vi "Actor Core.vi"(8 "error in":errorcluster, 11 "XY WFRM Plot in":refnum<class "XY WFRM Plot.lvclass">) -> (0 "error out":errorcluster, 3 "Actor out":refnum<class "Actor.lvclass">)   [LabVIEW 2020, in "XY WFRM Plot.lvclass"]
doc: "Plots listed TDMS data files"
uses:
  XY WFRM Plot.lvclass
  opt/github/LabActor/Template Module/Template Module.lvclass
  opt/github/LabActor/Plots/Plot/Plot.lvclass
  Applications/National Instruments/LabVIEW 2020 64-bit/vi.lib/ActorFramework/Actor/Actor.lvclass
  <vilib>/ActorFramework/Actor/Actor.lvclass
  Plot types.ctl
  XY WFRM Plot.lvclass/XY WFRM Plot.ctl
  Template Module/Template Module.lvclass/Template Module.ctl
  Plot/Plot.lvclass/Plot.ctl
  <vilib>/ActorFramework/Actor/Actor.lvclass/Actor.ctl
  <vilib>/ActorFramework/Message Enqueuer/Message Enqueuer.lvclass/Message Enqueuer.ctl
  XY WFRM Plot Messages/Set Plot Type Msg/Set Plot Type Msg.lvclass/Set Plot Type Msg.ctl
  Plot Messages/Write Files Msg/Write Files Msg.lvclass/Write Files Msg.ctl
  Plot Messages/Write Keep # of preceding files Msg/Write File history depth Msg.lvclass/Write File history depth Msg.ctl
  Controllers/Application Controller Messages/Open TDMS Properties Msg/Open TDMS Properties Msg.lvclass/Open TDMS Properties Msg.ctl
  Template Module/Read stop event.vi
  Read Plot type.vi
  Plot/WriteFile history depth.vi
  <vilib>/ActorFramework/Message Enqueuer/Init from Existing Queue.vi
  <vilib>/ActorFramework/Message Enqueuer/Enqueue.vi
  XY WFRM Plot Messages/Set Plot Type Msg/Set Plot Type Msg.lvclass
  Applications/National Instruments/LabVIEW 2020 64-bit/vi.lib/ActorFramework/Message/Message.lvclass
  Plot Messages/Replot Msg/Replot Msg.lvclass
  Plot Messages/Write Files Msg/Write Files Msg.lvclass
  <vilib>/ActorFramework/Stop Msg/Stop Msg.lvclass
  Plot Messages/Write Keep # of preceding files Msg/Write File history depth Msg.lvclass
  Controllers/Application Controller Messages/Open TDMS Properties Msg/Open TDMS Properties Msg.lvclass
  <vilib>/ActorFramework/Message Priority Queue/Priority Enqueue.vi
  Plot/Plot.lvclass
  <vilib>/ActorFramework/Message Enqueuer/Message Enqueuer.lvclass
panel:
  in  "Open properties":bool
  in  "File history depth":i32=2
  out "Waveform Plot":waveform(sgl)[](graph)
  in  "Y column(s)":i32[](listbox)=[1]
  in  "X column":i32(listbox)
  in  "File(s)":path[](array[path])
  out "XY Plot":cluster{"Y":dbl[], "Y":dbl[]}[](graph)
  in  "Plot type":enum32{"X-Y Plot", "Waveform Plot"}(tab)
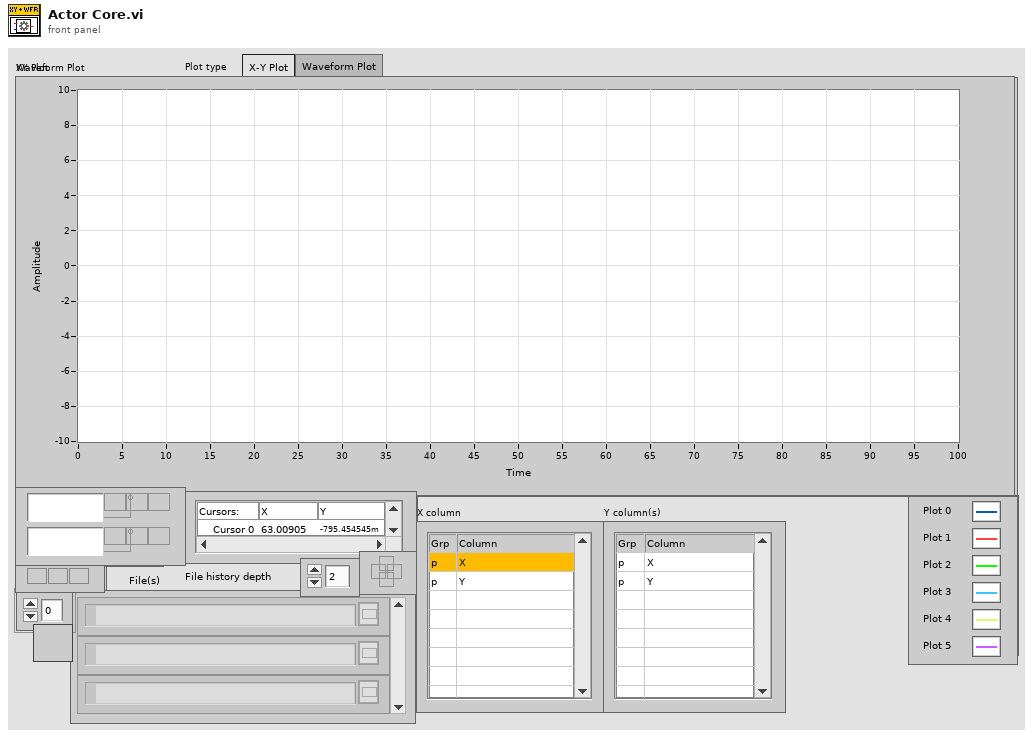
[diagram p1: front panel]
types:
  T1 = typedef "Plot types.ctl" = enum16{"Waveform Plot", "XY Plot", "Full XY"}
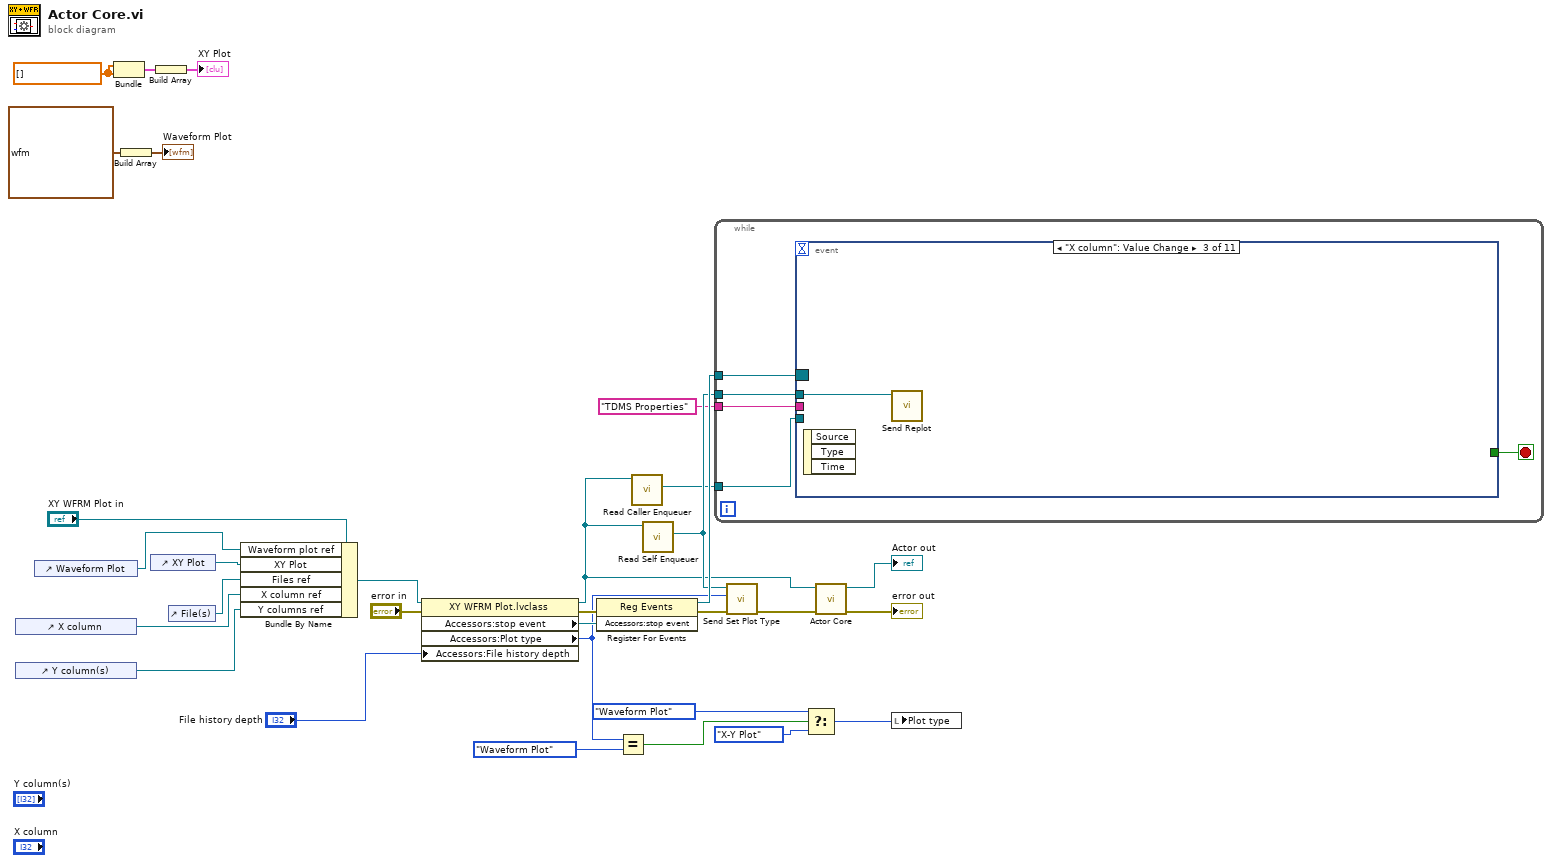
[diagram p0: block diagram]
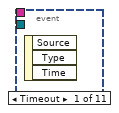
[diagram p2: hidden frame]
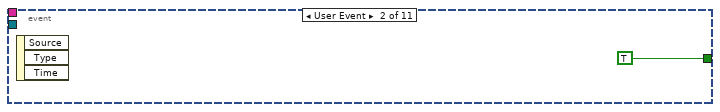
[diagram p3: hidden frame]
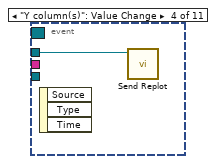
[diagram p4: hidden frame]
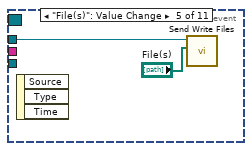
[diagram p5: hidden frame]
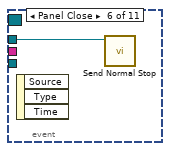
[diagram p6: hidden frame]
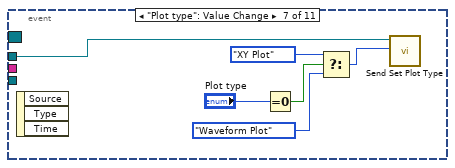
[diagram p7: hidden frame]
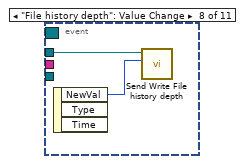
[diagram p8: hidden frame]
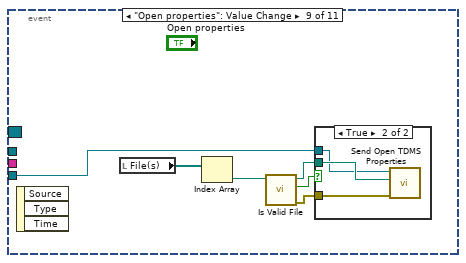
[diagram p9: hidden frame]
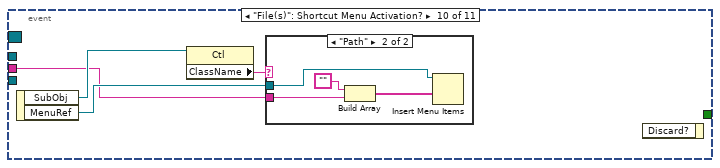
[diagram p11: hidden frame]
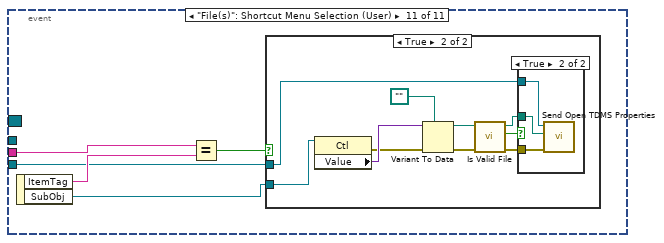
[diagram p13: hidden frame]
diagram:
  w18 = dbl[] [] ("Y")
  n1 = control-ref of="X column"() -> (w24:refnum<vi>)
  n2 = control-ref of="Y column(s)"() -> (w25:refnum<vi>)
  n3 = control-ref of="Waveform Plot"() -> (w15:refnum<vi>)
  n4 = Bundle("Y"=w18, "Y"=w18) -> (w17:cluster{"Y":dbl[], "Y":dbl[]})  [unwired: 1 in]
  n5 = Build Array(waveform(sgl) {"t0"=timestamp(0 s since 1904-01-01), "dt"=1.0, "Y"=[]} ("Waveform")) -> (→"Waveform Plot":waveform(sgl)[])
  n6 = control-ref of="XY Plot"() -> (w27:refnum<vi>)
  n7 = Build Array(w17) -> (→"XY Plot":cluster{"Y":dbl[], "Y":dbl[]}[])
  n8 = control-ref of="File(s)"() -> (w26:refnum<vi>)
  n9 = Bundle By Name(cluster="XY WFRM Plot in", "Waveform plot ref"=w15, "XY Plot"=w27, "Files ref"=w26, "X column ref"=w24, "Y columns ref"=w25) -> (w28:refnum<class "XY WFRM Plot.lvclass">)
  n10 = property class="XY WFRM Plot.lvclass"(reference=w28, error in="error in", "Accessors:File history depth"="File history depth") -> (reference out=w3:refnum<class "XY WFRM Plot.lvclass">, error out=w21:errorcluster, "Accessors:stop event"=w23:refnum<user-event>, "Accessors:Plot type"=w8:T1)
  n11 = register-events(error in=w21, w23) -> (reference out=w22:refnum<event-registration>, error out=w12:errorcluster)  [unwired: 1 in]
  n12 = Equal?(x=w8, y=Plot_types."Waveform Plot" ("Plot type")) -> (x = y?=w13:bool)
  n13 = call <vilib>:"Read Caller Enqueuer.vi"("Actor"=w3) -> ("Caller Enqueuer"=w2:refnum<class "Message Enqueuer.lvclass">)  [unwired: 10 in]
  n14 = call <vilib>:"Read Self Enqueuer.vi"("Actor"=w3) -> ("Self Enqueuer"=w10:refnum<class "Message Enqueuer.lvclass">)  [unwired: 10 in]
  n15 = while {
    tunnel: w22 -> [w36]
    tunnel: w10 -> [w34]
    tunnel: w2 -> [w33]
    tunnel: "TDMS Properties" -> [w32]
    stop <- w35 stop-if-true
    n16 = event shown="[2] \"X column\": Value Change" {
      selector: w36 -> [_ _ _ _ _ _ _ _ _ _ _]
      dyn-events: _ -> [_ _ _ _ _ _ _ _ _ _ _]
      timeout: _ -> [_ _ _ _ _ _ _ _ _ _ _]
      tunnel: [_ TRUE _ _ _ _ _ _ _ _ _] -> w35
      tunnel: w34 -> [_ _ w38 w39 w41 w42 w47 w50 _ _ _]
      tunnel: w33 -> [_ _ _ _ _ _ _ _ w52 _ w68]
      tunnel: w32 -> [_ _ _ _ _ _ _ _ _ w60 w71]
      event Timeout {
        n17 = event-data() -> ()  [unwired: 1 in, 3 out]
      }
      event User Event {
        n18 = event-data() -> ()  [unwired: 1 in, 3 out]
      }
      event "X column": Value Change {
        n19 = event-data() -> ()  [unwired: 1 in, 3 out]
        n20 = call "Send Replot.vi"("Message Enqueuer"=w38) -> ()  [unwired: 9 in, 2 out]
      }
      event "Y column(s)": Value Change {
        n21 = event-data() -> ()  [unwired: 1 in, 3 out]
        n22 = call "Send Replot.vi"("Message Enqueuer"=w39) -> ()  [unwired: 9 in, 2 out]
      }
      event "File(s)": Value Change {
        n23 = event-data() -> ()  [unwired: 1 in, 3 out]
        n24 = call "Send Write Files.vi"("Files"="File(s)", "Message Enqueuer"=w41) -> ()  [unwired: 8 in, 2 out]
      }
      event Panel Close {
        n25 = event-data() -> ()  [unwired: 1 in, 3 out]
        n26 = call <vilib>:"Send Normal Stop.vi"("Message Enqueuer"=w42) -> ()  [unwired: 10 in, 1 out]
      }
      event "Plot type": Value Change {
        n27 = event-data() -> ()  [unwired: 1 in, 3 out]
        n28 = Equal To 0?(x="Plot type") -> (x = 0?=w46:bool)
        n29 = Select(t=Plot_types."XY Plot" ("Plot type"), s=w46, f=Plot_types."Waveform Plot" ("Plot type")) -> (s? t:f=w45:T1)
        n30 = call "Send Set Plot Type.vi"("Plot type"=w45, "Message Enqueuer"=w47) -> ()  [unwired: 8 in, 2 out]
      }
      event "File history depth": Value Change {
        n31 = event-data() -> ("NewVal"=w49:i32)  [unwired: 1 in, 2 out]
        n32 = call "Send Write File history depth.vi"("File history depth"=w49, "Message Enqueuer"=w50) -> ()  [unwired: 8 in, 2 out]
      }
      event "Open properties": Value Change {
        n33 = event-data() -> ()  [unwired: 1 in, 3 out]
        n34 = local read "File(s)"() -> (w56:path[])
        n35 = Index Array(array=w56) -> (element=w55:path)  [unwired: 1 in]
        n36 = call "Is Valid File.vi"("File"=w55) -> ("Error Out"=w51:errorcluster, "Valid file"=w54:bool, "File out"=w53:path)  [unwired: 8 in]
        n37 = case shown="True" w54 {
          tunnel: w53 -> [_ w59]
          tunnel: w52 -> [_ w58]
          tunnel: w51 -> [_ w57]
          frame False {
          }
          frame True {
            n38 = call "Send Open TDMS Properties.vi"("error in (no error)"=w57, "File"=w59, "Message Enqueuer"=w58) -> ()  [unwired: 7 in, 2 out]
          }
        }
      }
      event "File(s)": Shortcut Menu Activation? {
        n39 = event-data() -> ("SubObj"=w63:refnum<vi>, "MenuRef"=w61:refnum<k9>)  [unwired: 1 in]
        n40 = property class="Ctl"(reference=w63) -> ("ClassName"=w62:string)  [unwired: 1 in, 2 out]
        n41 = case shown="\"Path\"" w62 {
          tunnel: w61 -> [_ w67]
          tunnel: w60 -> [_ w65]
          frame "False", Default {
          }
          frame "Path" {
            n42 = Build Array("", w65) -> (w66:string[])
            n43 = Insert Menu Items(7:w66, 9:w67) -> ()  [unwired: 4 in, 3 out]
          }
        }
        n44 = event-data() -> ()  [unwired: 2 in, 1 out]
      }
      event "File(s)": Shortcut Menu Selection (User) {
        n45 = event-data() -> ("ItemTag"=w72:string, "SubObj"=w69:refnum<vi>)  [unwired: 1 in]
        n46 = Equal?(x=w71, y=w72) -> (x = y?=w70:bool)
        n47 = case shown="True" w70 {
          tunnel: w69 -> [_ w80]
          tunnel: w68 -> [_ w74]
          frame False {
          }
          frame True {
            n48 = property class="Ctl"(reference=w80) -> (error out=w73:errorcluster, "Value"=w81:variant)  [unwired: 1 in, 1 out]
            n49 = Variant To Data(error in=w73, type=path "", Variant=w81) -> (data=w75:path, error out=w76:errorcluster)
            n50 = call "Is Valid File.vi"("Error In"=w76, "File"=w75) -> ("Error Out"=w77:errorcluster, "Valid file"=w79:bool, "File out"=w78:path)  [unwired: 7 in]
            n51 = case shown="True" w79 {
              tunnel: w78 -> [_ w85]
              tunnel: w77 -> [_ w84]
              tunnel: w74 -> [_ w83]
              frame False {
              }
              frame True {
                n52 = call "Send Open TDMS Properties.vi"("error in (no error)"=w84, "File"=w85, "Message Enqueuer"=w83) -> ()  [unwired: 7 in, 2 out]
              }
            }
          }
        }
      }
    }
  }
  n53 = call "Send Set Plot Type.vi"("error in (no error)"=w12, "Plot type"=w8, "Message Enqueuer"=w10) -> ("error out"=w11:errorcluster)  [unwired: 7 in, 1 out]
  n54 = Select(t=enum32{"X-Y Plot", "Waveform Plot"}."Waveform Plot" ("Plot type"), s=w13, f=enum32{"X-Y Plot", "Waveform Plot"}."X-Y Plot" ("Plot type")) -> (s? t:f=w9:enum32{"X-Y Plot", "Waveform Plot"})
  n55 = call-parent "Actor Core.vi"("error in"=w11, "Measure Object in"=w3) -> ("error out"=→"error out":errorcluster, "Actor out"=→"Actor out":refnum<class "Actor.lvclass">)  [unwired: 8 in]
  n56 = local write "Plot type"(w9) -> ()
